vi "6220_SaveToTDMS.vi"(10 "数据":T1={"时间"=timestamp(3515985789.500352 s since 1904-01-01), "陪试轴承润滑单元出油温度1"=array[32000 elements], "陪试轴承润滑单元出油温度2"=array[32000 elements], "轴承外圈温度"=array[32000 elements], "出油温度"=array[32000 elements], "摩擦力1"=array[32000 elements], "摩擦力2"=array[32000 elements], "径向油缸力"=array[80000 elements], "轴向油缸力"=array[80000 elements], "转速"=array[80000 elements]}, 11 "文件名":string="data") -> (3 "错误输出":errorcluster)   [LabVIEW 2014]
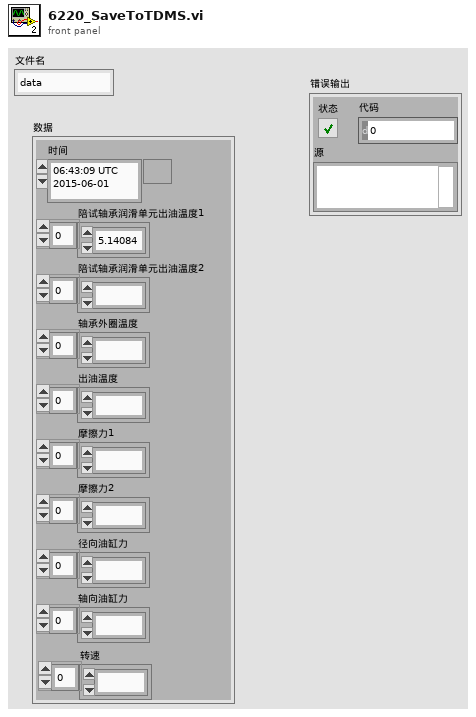
[diagram p1: front panel]
types:
  T1 = cluster{"时间":timestamp, "陪试轴承润滑单元出油温度1":sgl[], "陪试轴承润滑单元出油温度2":sgl[], "轴承外圈温度":sgl[], "出油温度":sgl[], "摩擦力1":sgl[], "摩擦力2":sgl[], "径向油缸力":sgl[], "轴向油缸力":sgl[], "转速":sgl[]}
  T2 = cluster{string, string, string, string, string, string, string, string, string}
  T3 = enum16{"open", "open or create", "create or replace", "create", "open (read-only)"}
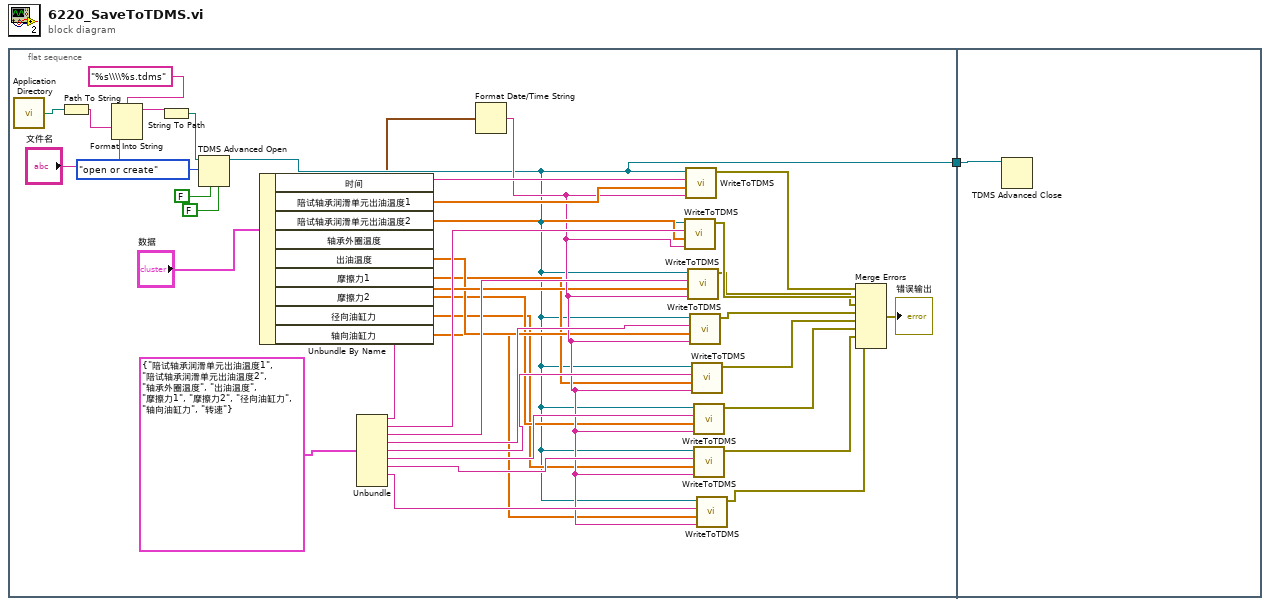
[diagram p0: block diagram]
diagram:
  n1 = flat-sequence {
    tunnel: [w7] -> w1
    tunnel: w1 -> [w41]
    frame #0 {
      n2 = call <vilib>:"Application Directory.vi"() -> ("Application Directory"=w38:path)
      n3 = Path To String(path=w38) -> (string=w39:string)
      n4 = Format Into String(format string="%s\\\\%s.tdms", w39, "文件名") -> (resulting string=w40:string)  [unwired: 2 in, 1 out]
      n5 = String To Path(string=w40) -> (path=w36:path)
      n6 = TDMS Advanced Open(4:FALSE ("启用异步？(T)"), 6:FALSE ("禁用缓冲？(T)"), 10:T3."open or create" ("操作(0:open)"), 11:w36) -> (3:w7:refnum<k34>)  [unwired: 1 in, 2 out]
      n7 = Unbundle By Name("数据") -> ("时间"=w5:timestamp, "陪试轴承润滑单元出油温度1"=w32:sgl[], "陪试轴承润滑单元出油温度2"=w24:sgl[], "轴承外圈温度"=w22:sgl[], "出油温度"=w21:sgl[], "摩擦力1"=w20:sgl[], "摩擦力2"=w19:sgl[], "径向油缸力"=w18:sgl[], "轴向油缸力"=w17:sgl[])
      n8 = Unbundle(T2 {"陪试轴承润滑单元出油温度1", "陪试轴承润滑单元出油温度2", "轴承外圈温度", "出油温度", "摩擦力1", "摩擦力2", "径向油缸力", "轴向油缸力", "转速"} ("通道名")) -> (w33:string, w31:string, w30:string, w29:string, w28:string, w27:string, w26:string, w25:string)  [unwired: 1 out]
      n9 = Format Date/Time String(seconds (now)=w5) -> (date/time string=w23:string)  [unwired: 2 in]
      n10 = call "WriteToTDMS.vi"("组名称（未命名）"=w23, "数据"=w24, "通道名"=w31, "tdms文件"=w7) -> ("错误输出"=w15:errorcluster)  [unwired: 7 in]
      n11 = call "WriteToTDMS.vi"("组名称（未命名）"=w23, "数据"=w32, "通道名"=w33, "tdms文件"=w7) -> ("错误输出"=w16:errorcluster)  [unwired: 7 in]
      n12 = call "WriteToTDMS.vi"("组名称（未命名）"=w23, "数据"=w22, "通道名"=w30, "tdms文件"=w7) -> ("错误输出"=w14:errorcluster)  [unwired: 7 in]
      n13 = call "WriteToTDMS.vi"("组名称（未命名）"=w23, "数据"=w21, "通道名"=w29, "tdms文件"=w7) -> ("错误输出"=w13:errorcluster)  [unwired: 7 in]
      n14 = call "WriteToTDMS.vi"("组名称（未命名）"=w23, "数据"=w20, "通道名"=w28, "tdms文件"=w7) -> ("错误输出"=w12:errorcluster)  [unwired: 7 in]
      n15 = call "WriteToTDMS.vi"("组名称（未命名）"=w23, "数据"=w19, "通道名"=w27, "tdms文件"=w7) -> ("错误输出"=w11:errorcluster)  [unwired: 7 in]
      n16 = call "WriteToTDMS.vi"("组名称（未命名）"=w23, "数据"=w18, "通道名"=w26, "tdms文件"=w7) -> ("错误输出"=w10:errorcluster)  [unwired: 7 in]
      n17 = call "WriteToTDMS.vi"("组名称（未命名）"=w23, "数据"=w17, "通道名"=w25, "tdms文件"=w7) -> ("错误输出"=w9:errorcluster)  [unwired: 7 in]
      n18 = Merge Errors(w16, w15, w14, w13, w12, w11, w10, w9) -> (→"错误输出":errorcluster)
    }
    frame #1 {
      n19 = TDMS Advanced Close(11:w41) -> ()  [unwired: 3 in, 2 out]
    }
  }
